vi "UI_Show_Hide_Clusters.vi"(8 "error in (no error)":errorcluster, 10 "Enable ?":bool, 11 "Clusters":refnum<vi>[](array[refnum])) -> (0 "error out":errorcluster caption="sortie d'erreur")   [LabVIEW 2018]
doc: "This VI shows or hides a list of Clusters."
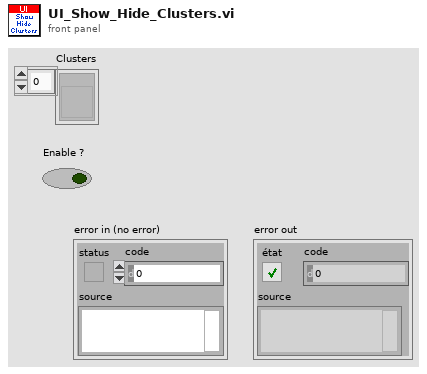
[diagram p1: front panel]
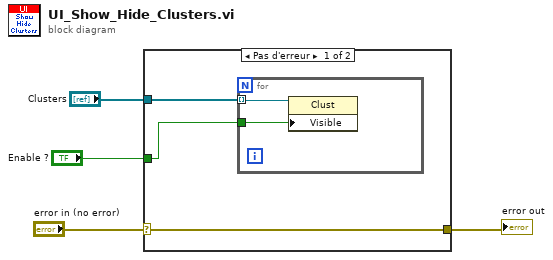
[diagram p0: block diagram]
diagram:
  n1 = case shown="Pas d'erreur" "error in (no error)" {
    selector: "error in (no error)" -> [w6 w10]
    tunnel: "Clusters" -> [w7 _]
    tunnel: "Enable ?" -> [w5 _]
    tunnel: [w6 w10] -> w1
    frame No Error {
      n2 = for {
        tunnel: w7 -> [w9] mode=indexing
        tunnel: w5 -> [w8]
        n3 = property class="Clust"(reference=w9, "Visible"=w8) -> ()  [unwired: 1 in, 2 out]
      }
    }
    frame Error {
    }
  }
  "error out" <- w1
